vi "osa_get LUT.vi"(2 "sensor map settings":cluster{"OSB index":u8[], "display index":i32[]}={"OSB index"=[1, 2, 3, 4, 5, 6, 7], "display index"=[26, 22, 18, 14, 10, 6, 2]}) -> (6 "sensor LUT":variant)   [LabVIEW 2021]
panel:
  # "OSA subVI: get OSB and sensor LUT (lookup table)"
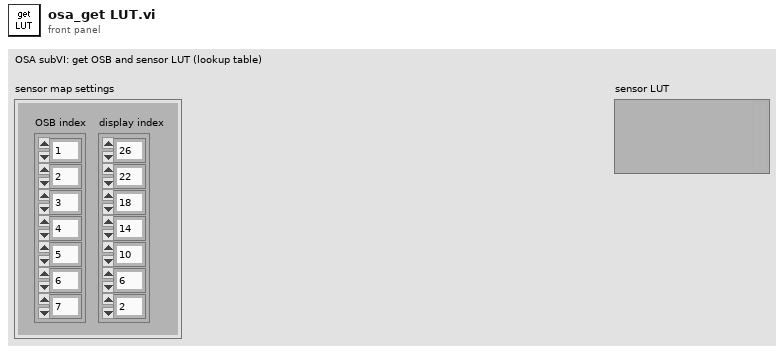
[diagram p1: front panel]
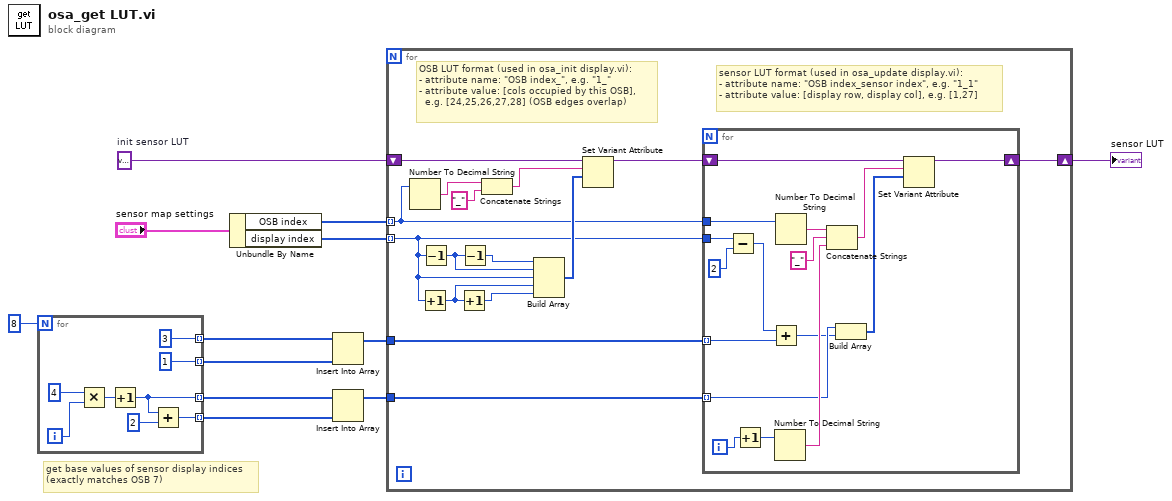
[diagram p0: block diagram]
diagram:
  w9 = variant  # init sensor LUT
  # "get base values of sensor display indices\n(exactly matches OSB 7)"
  n1 = for {
    N: 8 -> [_]
    tunnel: [w16] -> w7 mode=indexing
    tunnel: [w15] -> w6 mode=indexing
    tunnel: [3] -> w5 mode=indexing
    tunnel: [1] -> w4 mode=indexing
    i -> [w20]
    n2 = Multiply(x=4, y=w20) -> (x*y=w18:i32)
    n3 = Increment(x=w18) -> (x+1=w16:i32)
    n4 = Add(x=w16, y=2) -> (x+y=w15:i32)
  }
  n5 = Unbundle By Name("sensor map settings") -> ("OSB index"=w11:u8[], "display index"=w10:i32[])
  n6 = Insert Into Array(array=w5, new element=w4) -> (w3:i32[])  [unwired: 1 in]
  n7 = Insert Into Array(array=w7, new element=w6) -> (w2:i32[])  [unwired: 1 in]
  n8 = for {
    tunnel: w11 -> [w27] mode=indexing
    tunnel: w10 -> [w25] mode=indexing
    shift-right: [w26] -> w1
    shift-left: w9 -> [w35]
    tunnel: w3 -> [w29]
    tunnel: w2 -> [w28]
    # "sensor LUT format (used in osa_update display.vi):\n- attribute name: \"OSB index_sensor index\", e.g. \"1_1\"\n- attribute value: [display row, display col], e.g. [1,27]"
    # "OSB LUT format (used in osa_init display.vi):\n- attribute name: \"OSB index_\", e.g. \"1_\"\n- attribute value: [cols occupied by this OSB],\n  e.g. [24,25,26,27,28] (OSB edges overlap)"
    n9 = Number To Decimal String(number=w27) -> (decimal integer string=w34:string)  [unwired: 1 in]
    n10 = Increment(x=w25) -> (x+1=w22:i32)
    n11 = Decrement(x=w25) -> (x-1=w24:i32)
    n12 = Increment(x=w22) -> (x+1=w21:i32)
    n13 = Decrement(x=w24) -> (x-1=w23:i32)
    n14 = Concatenate Strings(w34, "_") -> (w32:string)
    n15 = Build Array(w23, w24, w25, w22, w21) -> (w31:i32[])
    n16 = Set Variant Attribute(Variant=w35, name=w32, value=w31) -> (Variant out=w30:variant)  [unwired: 1 in, 2 out]
    n17 = for {
      shift-right: [w50] -> w26
      shift-left: w30 -> [w51]
      tunnel: w29 -> [w39] mode=indexing
      tunnel: w28 -> [w38] mode=indexing
      tunnel: w27 -> [w49]
      tunnel: w25 -> [w42]
      i -> [w46]
      n18 = Subtract(x=w42, y=2) -> (x-y=w40:i32)
      n19 = Increment(x=w46) -> (x+1=w45:i32)
      n20 = Add(x=w40, y=w39) -> (x+y=w37:i32)
      n21 = Number To Decimal String(number=w45) -> (decimal integer string=w44:string)  [unwired: 1 in]
      n22 = Number To Decimal String(number=w49) -> (decimal integer string=w48:string)  [unwired: 1 in]
      n23 = Concatenate Strings(w48, "_", w44) -> (w43:string)
      n24 = Build Array(w38, w37) -> (w36:i32[])
      n25 = Set Variant Attribute(Variant=w51, name=w43, value=w36) -> (Variant out=w50:variant)  [unwired: 1 in, 2 out]
    }
  }
  "sensor LUT" <- w1
